vi "HFRR ADV v07.vi"() -> ()   [LabVIEW 2025] (continued)
                frame 81 {
                  n3117 = property on="Air Temperature  ( °C )" class="XYGraph (strict)"("Y Scale.Name Label.Text"=w4156) -> ()  [unwired: 2 in, 2 out]
                }
                frame 82 {
                  n3118 = local write "S 84"(w4157) -> ()
                }
                frame 83 {
                  n3119 = local write "S 85"(w4158) -> ()
                }
                frame 84 {
                  n3120 = local write "S 86"(w4159) -> ()
                }
                frame 85 {
                  n3121 = local write "S 87"(w4160) -> ()
                }
                frame 86 {
                  n3122 = local write "S 88"(w4161) -> ()
                }
                frame 87 {
                }
                frame 88 {
                  n3123 = local write "S 90"(w4163) -> ()
                }
                frame 89 {
                  n3124 = local write "S 91"(w4164) -> ()
                }
                frame 90 {
                  n3125 = local write "S 92"(w4165) -> ()
                }
                frame 91 {
                  n3126 = local write "S 93"(w4166) -> ()
                }
                frame 92 {
                  n3127 = local write "S 94"(w4167) -> ()
                }
                frame 93 {
                  n3128 = local write "S 95"(w4168) -> ()
                }
                frame 94 {
                  n3129 = local write "S 96"(w4169) -> ()
                }
                frame 95 {
                  n3130 = local write "S 97"(w4170) -> ()
                }
                frame 96 {
                  n3131 = local write "S 98"(w4171) -> ()
                }
                frame 97 {
                  n3132 = local write "S 99"(w4172) -> ()
                }
                frame 98 {
                  n3133 = local write "S 100"(w4173) -> ()
                }
                frame 99 {
                  n3134 = local write "S 101"(w4174) -> ()
                }
                frame 100 {
                  n3135 = local write "S 102"(w4175) -> ()
                }
                frame 101 {
                  n3136 = local write "S 103"(w4176) -> ()
                }
                frame 102 {
                  n3137 = local write "S 104"(w4177) -> ()
                }
                frame 103 {
                  n3138 = local write "S 105"(w4178) -> ()
                }
                frame 104 {
                  n3139 = local write "S 106"(w4179) -> ()
                }
                frame 105 {
                }
                frame 106 {
                  n3140 = property on="OK Button 17" class="Bool (strict)"("Boolean Text.Text"=w4180) -> ()  [unwired: 2 in, 2 out]
                }
                frame 107 {
                  n3141 = property on="OK Button 16" class="Bool (strict)"("Boolean Text.Text"=w4181) -> ()  [unwired: 2 in, 2 out]
                }
                frame 108 {
                  n3142 = property on="TITTLE" class="Str"("Caption.Text"=w4182) -> ()  [unwired: 2 in, 2 out]
                }
                frame 109 {
                  "String 30" <- w4183
                }
                frame 110 {
                  n3143 = property on="Test Date" class="Str"("Caption.Text"=w4184) -> ()  [unwired: 2 in, 2 out]
                  "String 31" <- w4184
                }
                frame 111 {
                  n3144 = property on="Sample ID" class="Str"("Caption.Text"=w4185) -> ()  [unwired: 2 in, 2 out]
                  "String 32" <- w4185
                }
                frame 112 {
                  n3145 = property on="Tested by" class="Str"("Caption.Text"=w4186) -> ()  [unwired: 2 in, 2 out]
                  "String 33" <- w4186
                }
                frame 113 {
                  n3146 = property on="System Configured Printers 2" class="Arr (strict)"("Caption.Text"=w4187) -> ()  [unwired: 2 in, 2 out]
                }
                frame 114 {
                  n3147 = property on="Selected Printer" class="Str"("Caption.Text"=w4188) -> ()  [unwired: 2 in, 2 out]
                }
                frame 115 {
                  n3148 = property on="Select Printer 3" class="DigNum (strict)"("Caption.Text"=w4189) -> ()  [unwired: 2 in, 2 out]
                }
                frame 116 {
                  n3149 = property on="Print" class="Bool (strict)"("Boolean Text.Text"=w4190) -> ()  [unwired: 2 in, 2 out]
                }
                frame 117 {
                  "String 41" <- w4191
                }
                frame 118 {
                  n3150 = property on="tested by" class="Str"("Caption.Text"=w4192) -> ()  [unwired: 2 in, 2 out]
                }
                frame 119 {
                }
                frame 120 {
                  n3151 = property on="Export" class="Bool (strict)"("Boolean Text.Text"=w4193) -> ()  [unwired: 2 in, 2 out]
                }
                frame 121 {
                  n3152 = property on="TEMP INTERCEPT:" class="DigNum (strict)"("Caption.Text"=w4194) -> ()  [unwired: 2 in, 2 out]
                }
                frame 122 {
                  n3153 = property on="AIR TEMP INTERCEPT:" class="DigNum (strict)"("Caption.Text"=w4195) -> ()  [unwired: 2 in, 2 out]
                }
                frame 123 {
                  n3154 = property on="Select File Type" class="Enum (strict)"("Caption.Text"=w4196) -> ()  [unwired: 2 in, 2 out]
                }
                frame 124 {
                  n3155 = property on="s.NO" class="Str"("Caption.Text"=w4197) -> ()  [unwired: 2 in, 2 out]
                  "String 45" <- w4197
                }
                frame 125 {
                  n3156 = property on="trip1 8" class="Bool (strict)"("Boolean Text.Text"=w4198) -> ()  [unwired: 2 in, 2 out]
                }
                frame 126, Default {
                }
              }
            }
          }
          frame #1 {
            w4206 = TRUE ("Visible")
            n3157 = local read "S 91"() -> (w4223:string)
            n3158 = local read "S 90"() -> (w4222:string)
            n3159 = local read "S 88"() -> (w4221:string)
            n3160 = property on="File Path" class="Path"("Caption.Text"=w4222) -> ()  [unwired: 2 in, 2 out]
            n3161 = property on="SrvM CP" class="Bool (strict)"("Boolean Text.Text"=w4221) -> ()  [unwired: 2 in, 2 out]
            n3162 = local read "S 71"() -> (w4216:string)
            n3163 = local read "S 86"() -> (w4218:string)
            n3164 = local read "S 85"() -> (w4219:string)
            n3165 = local read "S 87"() -> (w4217:string)
            n3166 = local read "S 84"() -> (w4220:string)
            n3167 = local read "S 103"() -> (w4205:string)
            n3168 = local read "S 104"() -> (w4204:string)
            n3169 = property on="ENTER THE NEW PASSWORD" class="Str"("Caption.Text"=w4217) -> ()  [unwired: 2 in, 2 out]
            n3170 = property on="Password" class="Str"("Caption.Text"=w4219) -> ()  [unwired: 2 in, 2 out]
            n3171 = property on="ENTER CURRENT PASSWORD" class="Str"("Caption.Text"=w4218) -> ()  [unwired: 2 in, 2 out]
            n3172 = property on="EDIT" class="Bool (strict)"("Boolean Text.Text"=w4216) -> ()  [unwired: 2 in, 2 out]
            n3173 = property on="SAVE" class="Bool (strict)"("Boolean Text.Text"=w4220) -> ()  [unwired: 2 in, 2 out]
            n3174 = Build Array(w4205, w4204) -> (w4203:string[])
            n3175 = property on="Heater Button" class="Bool (strict)"("Strings [4]"=w4203) -> ()  [unwired: 2 in, 2 out]
            n3176 = property on="CH-HUMIDITY WET" class="DigNum (strict)"("Caption.Size to Text?"=w4206) -> ()  [unwired: 2 in, 2 out]
            n3177 = property on="CH-HUMIDITY DRY" class="DigNum (strict)"("Caption.Size to Text?"=w4206) -> ()  [unwired: 2 in, 2 out]
            n3178 = property on="CH-POWER -" class="DigNum (strict)"("Caption.Size to Text?"=w4206) -> ()  [unwired: 2 in, 2 out]
            n3179 = property on="CH-HEATER" class="DigNum (strict)"("Caption.Size to Text?"=w4206) -> ()  [unwired: 2 in, 2 out]
            n3180 = property on="CH-POWER +" class="DigNum (strict)"("Caption.Size to Text?"=w4206) -> ()  [unwired: 2 in, 2 out]
            n3181 = local read "S 92"() -> (w4215:string)
            n3182 = local read "S 93"() -> (w4214:string)
            n3183 = local read "S 105"() -> (w4201:string)
            n3184 = local read "S 106"() -> (w4200:string)
            n3185 = Build Array(w4215, w4214) -> ()  [unwired: 1 out]
            n3186 = Build Array(w4201, w4200) -> (w4202:string[])
            n3187 = local read "S 95"() -> (w4212:string)
            n3188 = local read "S 94"() -> (w4213:string)
            n3189 = local read "bs"() -> (w4228:string)
            n3190 = local read "as"() -> (w4229:string)
            n3191 = property on="Humidity" class="Bool (strict)"("Strings [4]"=w4202) -> ()  [unwired: 2 in, 2 out]
            n3192 = Concatenate Strings(w4228, "\r", w4229) -> ()  [unwired: 1 out]
            n3193 = property on="STROKE GAIN :" class="DigNum (strict)"("Caption.Text"=w4212) -> ()  [unwired: 2 in, 2 out]
            n3194 = property on="DISPLACEMENT :" class="DigNum (strict)"("Caption.Text"=w4213) -> ()  [unwired: 2 in, 2 out]
            n3195 = property on="Rh After" class="DigNum (strict)"("Caption.Size to Text?"=TRUE ("Caption.Size to Text")) -> ()  [unwired: 2 in, 2 out]
            n3196 = local read "S 48"() -> (w4252:string)
            n3197 = local read "S 50"() -> (w4250:string)
            n3198 = local read "S 51"() -> (w4249:string)
            n3199 = local read "S 49"() -> (w4251:string)
            n3200 = local read "S 52"() -> (w4248:string)
            n3201 = local read "as"() -> (w4233:string)
            n3202 = local read "bs"() -> (w4234:string)
            n3203 = local read "S 56"() -> (w4247:string)
            n3204 = local read "S 57"() -> (w4246:string)
            n3205 = local read "S 58"() -> (w4245:string)
            n3206 = local read "S 59"() -> (w4244:string)
            n3207 = property on="OPEN" class="Bool (strict)"("Boolean Text.Text"=w4248) -> ()  [unwired: 2 in, 2 out]
            n3208 = property on="OPEN 1" class="Bool (strict)"("Boolean Text.Text"=w4252) -> ()  [unwired: 2 in, 2 out]
            n3209 = property on="OPEN 2" class="Bool (strict)"("Boolean Text.Text"=w4251) -> ()  [unwired: 2 in, 2 out]
            n3210 = property on="OPEN 3" class="Bool (strict)"("Boolean Text.Text"=w4250) -> ()  [unwired: 2 in, 2 out]
            n3211 = property on="OPEN 4" class="Bool (strict)"("Boolean Text.Text"=w4249) -> ()  [unwired: 2 in, 2 out]
            n3212 = Concatenate Strings(w4234, "\r", w4233) -> ()  [unwired: 1 out]
            n3213 = local read "S 102"() -> (w4207:string)
            n3214 = property on="КОФ1" class="DigNum (strict)"("Caption.Text"=w4247) -> ()  [unwired: 2 in, 2 out]
            n3215 = local read "S 98"() -> (w4211:string)
            n3216 = local read "S 99"() -> (w4210:string)
            n3217 = local read "S 100"() -> (w4209:string)
            n3218 = local read "S 101"() -> (w4208:string)
            n3219 = property on="КОФ2" class="DigNum (strict)"("Caption.Text"=w4246) -> ()  [unwired: 2 in, 2 out]
            n3220 = property on="КОФ3" class="DigNum (strict)"("Caption.Text"=w4245) -> ()  [unwired: 2 in, 2 out]
            n3221 = property on="КОФ4" class="DigNum (strict)"("Caption.Text"=w4244) -> ()  [unwired: 2 in, 2 out]
            n3222 = local read "bs"() -> (w4232:string)
            n3223 = local read "as"() -> (w4231:string)
            n3224 = property on="CH-POWER +" class="DigNum (strict)"("Caption.Text"=w4211) -> ()  [unwired: 2 in, 2 out]
            n3225 = property on="CH-POWER -" class="DigNum (strict)"("Caption.Text"=w4210) -> ()  [unwired: 2 in, 2 out]
            n3226 = property on="CH-HEATER" class="DigNum (strict)"("Caption.Text"=w4209) -> ()  [unwired: 2 in, 2 out]
            n3227 = property on="CH-HUMIDITY DRY" class="DigNum (strict)"("Caption.Text"=w4208) -> ()  [unwired: 2 in, 2 out]
            n3228 = property on="CH-HUMIDITY WET" class="DigNum (strict)"("Caption.Text"=w4207) -> ()  [unwired: 2 in, 2 out]
            n3229 = local read "S 60"() -> (w4243:string)
            n3230 = local read "S 54"() -> (w4253:string)
            n3231 = Concatenate Strings(w4232, "\r", w4231) -> ()  [unwired: 1 out]
            n3232 = Concatenate Strings(w4253, w4243) -> ()  [unwired: 1 out]
            n3233 = local read "S 77"() -> (→"String 43":string)
            n3234 = local read "S 76"() -> (w4226:string)
            n3235 = local read "S 78"() -> (w4225:string)
            n3236 = local read "S 71"() -> (w4237:string)
            n3237 = local read "S 66"() -> (w4242:string)
            n3238 = local read "S 67"() -> (w4241:string)
            n3239 = local read "S 68"() -> (w4240:string)
            n3240 = local read "S 69"() -> (w4239:string)
            n3241 = local read "S 70"() -> (w4238:string)
            n3242 = property on="AIR TEMP" class="DigNum (strict)"("Caption.Text"=w4225) -> ()  [unwired: 2 in, 2 out]
            n3243 = property on="Set Strk" class="DigNum (strict)"("Caption.Text"=w4226) -> ()  [unwired: 2 in, 2 out]
            n3244 = property on="FRIC. FORCE :" class="DigNum (strict)"("Caption.Text"=w4242) -> ()  [unwired: 2 in, 2 out]
            n3245 = property on="TEMPERATURE :" class="DigNum (strict)"("Caption.Text"=w4241) -> ()  [unwired: 2 in, 2 out]
            n3246 = property on="SPEED OUT:" class="DigNum (strict)"("Caption.Text"=w4240) -> ()  [unwired: 2 in, 2 out]
            n3247 = property on="AIR TEMPERATURE :" class="DigNum (strict)"("Caption.Text"=w4239) -> ()  [unwired: 2 in, 2 out]
            n3248 = property on="HUMIDITY:" class="DigNum (strict)"("Caption.Text"=w4238) -> ()  [unwired: 2 in, 2 out]
            n3249 = property on="EDIT" class="Bool (strict)"("Boolean Text.Text"=w4237) -> ()  [unwired: 2 in, 2 out]
            n3250 = local read "S 79"() -> (w4224:string)
          }
          frame #2 {
          }
        }
        n3251 = local write "Lan flag"(10.0 ("Lan flag")) -> ()
      }
      frame Enabled {
      }
    }
    n3252 = Wait (ms)(milliseconds to wait=u32 2000) -> ()  [unwired: 1 out]
    n3253 = local read "Quit"() -> (w4027:bool)
  }
  n3254 = disable-structure shown="Disabled" {
    frame Disabled {
      n3255 = while {
        tunnel: [w4255] -> _
        i -> [w4255]
        stop <- w4254 continue-if-true
        n3256 = Wait (ms)(milliseconds to wait=u32 50) -> ()  [unwired: 1 out]
        n3257 = stacked-sequence {
          frame #0 {
            # "Controls Text color"
            # "Controls BG color"
            n3258 = property on="FILE" class="Str"("Text.Text Colors:Text Color"="SC  Text") -> ()  [unwired: 2 in, 2 out]
            n3259 = property on="Fuel Discription :" class="Str"("Text.Text Colors:Text Color"="SC  Text") -> ()  [unwired: 2 in, 2 out]
            n3260 = property on="tested by" class="Str"("Text.Text Colors:Text Color"="SC  Text") -> ()  [unwired: 2 in, 2 out]
            n3261 = property on="Remarks :" class="Str"("Text.Text Colors:Text Color"="SC  Text") -> ()  [unwired: 2 in, 2 out]
            n3262 = property class="DigNum (strict)"("Numeric Text.Text Colors:BG Color"="NC BG") -> ()  [unwired: 2 in, 2 out]
            n3263 = property class="DigNum (strict)"("Numeric Text.Text Colors:BG Color"="NC BG") -> ()  [unwired: 2 in, 2 out]
            n3264 = property class="DigNum (strict)"("Numeric Text.Text Colors:BG Color"="NC BG") -> ()  [unwired: 2 in, 2 out]
            n3265 = property class="DigNum (strict)"("Numeric Text.Text Colors:BG Color"="NC BG") -> ()  [unwired: 2 in, 2 out]
            n3266 = property class="DigNum (strict)"("Numeric Text.Text Colors:BG Color"="NC BG") -> ()  [unwired: 2 in, 2 out]
            n3267 = property class="DigNum (strict)"("Numeric Text.Text Colors:BG Color"="NC BG") -> ()  [unwired: 2 in, 2 out]
            n3268 = property class="DigNum (strict)"("Numeric Text.Text Colors:BG Color"="NC BG") -> ()  [unwired: 2 in, 2 out]
            n3269 = property class="DigNum (strict)"("Numeric Text.Text Colors:BG Color"="NC BG") -> ()  [unwired: 2 in, 2 out]
            n3270 = property class="DigNum (strict)"("Numeric Text.Text Colors:BG Color"="NC BG") -> ()  [unwired: 2 in, 2 out]
            n3271 = property class="DigNum (strict)"("Numeric Text.Text Colors:BG Color"="NC BG") -> ()  [unwired: 2 in, 2 out]
            n3272 = property class="DigNum (strict)"("Numeric Text.Text Colors:BG Color"="NC BG") -> ()  [unwired: 2 in, 2 out]
            n3273 = property class="DigNum (strict)"("Numeric Text.Text Colors:BG Color"="NC BG") -> ()  [unwired: 2 in, 2 out]
            n3274 = property on="FILE" class="Str"("Text.Text Colors:BG Color"="SC BG 3") -> ()  [unwired: 2 in, 2 out]
            n3275 = property on="Fuel Discription :" class="Str"("Text.Text Colors:BG Color"="SC BG 3") -> ()  [unwired: 2 in, 2 out]
            n3276 = property on="tested by" class="Str"("Text.Text Colors:BG Color"="SC BG 3") -> ()  [unwired: 2 in, 2 out]
            n3277 = property on="Remarks :" class="Str"("Text.Text Colors:BG Color"="SC BG 3") -> ()  [unwired: 2 in, 2 out]
            n3278 = property class="DigNum (strict)"("Numeric Text.Text Colors:Text Color"="NC Text") -> ()  [unwired: 2 in, 2 out]
            n3279 = property class="DigNum (strict)"("Numeric Text.Text Colors:Text Color"="NC Text") -> ()  [unwired: 2 in, 2 out]
            n3280 = property class="DigNum (strict)"("Numeric Text.Text Colors:Text Color"="NC Text") -> ()  [unwired: 2 in, 2 out]
            n3281 = property class="DigNum (strict)"("Numeric Text.Text Colors:Text Color"="NC Text") -> ()  [unwired: 2 in, 2 out]
            n3282 = property class="DigNum (strict)"("Numeric Text.Text Colors:Text Color"="NC Text") -> ()  [unwired: 2 in, 2 out]
            n3283 = property class="DigNum (strict)"("Numeric Text.Text Colors:Text Color"="NC Text") -> ()  [unwired: 2 in, 2 out]
            n3284 = property class="DigNum (strict)"("Numeric Text.Text Colors:Text Color"="NC Text") -> ()  [unwired: 2 in, 2 out]
            n3285 = property class="DigNum (strict)"("Numeric Text.Text Colors:Text Color"="NC Text") -> ()  [unwired: 2 in, 2 out]
            n3286 = property class="DigNum (strict)"("Numeric Text.Text Colors:Text Color"="NC Text") -> ()  [unwired: 2 in, 2 out]
            n3287 = property class="DigNum (strict)"("Numeric Text.Text Colors:Text Color"="NC Text") -> ()  [unwired: 2 in, 2 out]
            n3288 = property class="DigNum (strict)"("Numeric Text.Text Colors:Text Color"="NC Text") -> ()  [unwired: 2 in, 2 out]
            n3289 = property class="DigNum (strict)"("Numeric Text.Text Colors:Text Color"="NC Text") -> ()  [unwired: 2 in, 2 out]
            n3290 = property class="DigNum (strict)"("Numeric Text.Text Colors:Text Color"="NI Text  2") -> ()  [unwired: 2 in, 2 out]
            n3291 = property class="DigNum (strict)"("Numeric Text.Text Colors:Text Color"="NI Text  2") -> ()  [unwired: 2 in, 2 out]
            n3292 = property class="DigNum (strict)"("Numeric Text.Text Colors:Text Color"="NI Text  2") -> ()  [unwired: 2 in, 2 out]
            n3293 = property class="DigNum (strict)"("Numeric Text.Text Colors:Text Color"="NI Text  2") -> ()  [unwired: 2 in, 2 out]
            n3294 = property class="DigNum (strict)"("Numeric Text.Text Colors:Text Color"="NI Text  2") -> ()  [unwired: 2 in, 2 out]
            n3295 = property class="DigNum (strict)"("Numeric Text.Text Colors:Text Color"="NI Text  2") -> ()  [unwired: 2 in, 2 out]
            n3296 = property class="DigNum (strict)"("Numeric Text.Text Colors:Text Color"="NI Text  2") -> ()  [unwired: 2 in, 2 out]
            n3297 = property class="DigNum (strict)"("Numeric Text.Text Colors:Text Color"="NI Text  2") -> ()  [unwired: 2 in, 2 out]
            n3298 = property class="DigNum (strict)"("Numeric Text.Text Colors:Text Color"="NI Text  2") -> ()  [unwired: 2 in, 2 out]
            n3299 = property class="DigNum (strict)"("Numeric Text.Text Colors:Text Color"="NI Text  2") -> ()  [unwired: 2 in, 2 out]
            n3300 = property class="DigNum (strict)"("Numeric Text.Text Colors:Text Color"="NI Text  2") -> ()  [unwired: 2 in, 2 out]
            n3301 = property class="DigNum (strict)"("Numeric Text.Text Colors:Text Color"="NI Text  2") -> ()  [unwired: 2 in, 2 out]
            n3302 = property class="DigNum (strict)"("Numeric Text.Text Colors:Text Color"="NI Text  2") -> ()  [unwired: 2 in, 2 out]
            n3303 = property class="DigNum (strict)"("Numeric Text.Text Colors:Text Color"="NI Text  2") -> ()  [unwired: 2 in, 2 out]
            n3304 = property class="DigNum (strict)"("Numeric Text.Text Colors:Text Color"="NI Text  2") -> ()  [unwired: 2 in, 2 out]
            n3305 = property on="Coefficient Of Friction" class="XYGraph (strict)"("Plot Area:Colors:FG Color"="GFG  2", "Plot Area:Colors:BG Color"="GBG   2") -> ()  [unwired: 2 in, 2 out]
            n3306 = property on="Humidity ( %RH )" class="XYGraph (strict)"("Plot Area:Colors:FG Color"="GFG  2", "Plot Area:Colors:BG Color"="GBG   2") -> ()  [unwired: 2 in, 2 out]
            n3307 = property on="Air Temperature  ( °C )" class="XYGraph (strict)"("Plot Area:Colors:FG Color"="GFG  2", "Plot Area:Colors:BG Color"="GBG   2") -> ()  [unwired: 2 in, 2 out]
            n3308 = property on="Sample Temperature ( °C )" class="XYGraph (strict)"("Plot Area:Colors:FG Color"="GFG  2", "Plot Area:Colors:BG Color"="GBG   2") -> ()  [unwired: 2 in, 2 out]
            n3309 = property class="DigNum (strict)"("Numeric Text.Text Colors:BG Color"="NI BG 2") -> ()  [unwired: 2 in, 2 out]
            n3310 = property class="DigNum (strict)"("Numeric Text.Text Colors:BG Color"="NI BG 2") -> ()  [unwired: 2 in, 2 out]
            n3311 = property class="DigNum (strict)"("Numeric Text.Text Colors:BG Color"="NI BG 2") -> ()  [unwired: 2 in, 2 out]
            n3312 = property class="DigNum (strict)"("Numeric Text.Text Colors:BG Color"="NI BG 2") -> ()  [unwired: 2 in, 2 out]
            n3313 = property class="DigNum (strict)"("Numeric Text.Text Colors:BG Color"="NI BG 2") -> ()  [unwired: 2 in, 2 out]
            n3314 = property class="DigNum (strict)"("Numeric Text.Text Colors:BG Color"="NI BG 2") -> ()  [unwired: 2 in, 2 out]
            n3315 = property class="DigNum (strict)"("Numeric Text.Text Colors:BG Color"="NI BG 2") -> ()  [unwired: 2 in, 2 out]
            n3316 = property class="DigNum (strict)"("Numeric Text.Text Colors:BG Color"="NI BG 2") -> ()  [unwired: 2 in, 2 out]
            n3317 = property class="DigNum (strict)"("Numeric Text.Text Colors:BG Color"="NI BG 2") -> ()  [unwired: 2 in, 2 out]
            n3318 = property class="DigNum (strict)"("Numeric Text.Text Colors:BG Color"="NI BG 2") -> ()  [unwired: 2 in, 2 out]
            n3319 = property class="DigNum (strict)"("Numeric Text.Text Colors:BG Color"="NI BG 2") -> ()  [unwired: 2 in, 2 out]
            n3320 = property class="DigNum (strict)"("Numeric Text.Text Colors:BG Color"="NI BG 2") -> ()  [unwired: 2 in, 2 out]
            n3321 = property class="DigNum (strict)"("Numeric Text.Text Colors:BG Color"="NI BG 2") -> ()  [unwired: 2 in, 2 out]
            n3322 = property class="DigNum (strict)"("Numeric Text.Text Colors:BG Color"="NI BG 2") -> ()  [unwired: 2 in, 2 out]
            n3323 = property class="DigNum (strict)"("Numeric Text.Text Colors:BG Color"="NI BG 2") -> ()  [unwired: 2 in, 2 out]
            n3324 = property class="Bool"("Colors [4]"="Boolean BC T & BG") -> ()  [unwired: 2 in, 2 out]
            n3325 = property on="Save & Continue" class="Bool (strict)"("Colors [4]"="Boolean BC T & BG") -> ()  [unwired: 2 in, 2 out]
            n3326 = property on="Heater Button" class="Bool (strict)"("Colors [4]"="Boolean BC T & BG") -> ()  [unwired: 2 in, 2 out]
            n3327 = property class="Bool"("Colors [4]"="Boolean BC T & BG") -> ()  [unwired: 2 in, 2 out]
            n3328 = property on="Humidity" class="Bool (strict)"("Colors [4]"="Boolean BC T & BG") -> ()  [unwired: 2 in, 2 out]
            n3329 = property class="Bool (strict)"("Colors [4]"="Boolean BC T & BG") -> ()  [unwired: 2 in, 2 out]
            n3330 = property on="RUN" class="Bool (strict)"("Colors [4]"="Boolean BC T & BG") -> ()  [unwired: 2 in, 2 out]
            n3331 = property on="trip1 8" class="Bool (strict)"("Colors [4]"="Boolean BC T & BG") -> ()  [unwired: 2 in, 2 out]
            n3332 = property class="Bool"("Colors [4]"="Boolean BC T & BG") -> ()  [unwired: 2 in, 2 out]
            n3333 = property class="Bool (strict)"("Colors [4]"="Boolean BC T & BG") -> ()  [unwired: 2 in, 2 out]
            n3334 = property on="OPEN 1" class="Bool (strict)"("Colors [4]"="Boolean BC T & BG 2") -> ()  [unwired: 2 in, 2 out]
            n3335 = property on="OPEN 2" class="Bool (strict)"("Colors [4]"="Boolean BC T & BG 2") -> ()  [unwired: 2 in, 2 out]
            n3336 = property on="OPEN 3" class="Bool (strict)"("Colors [4]"="Boolean BC T & BG 2") -> ()  [unwired: 2 in, 2 out]
            n3337 = property on="OPEN 4" class="Bool (strict)"("Colors [4]"="Boolean BC T & BG 2") -> ()  [unwired: 2 in, 2 out]
            n3338 = property on="OPEN" class="Bool (strict)"("Colors [4]"="Boolean BC T & BG 2") -> ()  [unwired: 2 in, 2 out]
            n3339 = property on="rstv2" class="Bool"("Colors [4]"="Boolean BC T & BG 2") -> ()  [unwired: 2 in, 2 out]
            n3340 = property on="RST CP" class="Bool"("Colors [4]"="Boolean BC T & BG 2") -> ()  [unwired: 2 in, 2 out]
            n3341 = property on="RSTV1 3" class="Bool"("Colors [4]"="Boolean BC T & BG 2") -> ()  [unwired: 2 in, 2 out]
            n3342 = property on="RSTV1 2" class="Bool"("Colors [4]"="Boolean BC T & BG 2") -> ()  [unwired: 2 in, 2 out]
          }
          frame #1 {
          }
        }
        n3343 = local read "Quit"() -> (w4254:bool)
      }
    }
    frame Enabled {
    }
  }
  n3344 = while {
    shift-right: [w4272] -> _
    shift-left: _ -> [w4273]
    shift-right: [w4270] -> _
    shift-left: T16 {"Read Heave and Surge"="", "Bytes at Heave Port"=0.0, "Heave and Surge COM Port:"="COM9", "Com Port 2"="COM7", "Residual Due"="", "Heave COM Status 2"=TRUE, "Heave COM Status"=TRUE, "Port 2"=TRUE, "Sway PPR"=6400.0, "Surge PPR"=6400.0, "Heave PPR"=6400.0, "Sway Pitch"=2.0, "Surge Pitch"=3.0, "Heave Pitch"=4.0, "Sway Pulses/mm"=320.0, "Surge Pulses/mm"=1600.0, "Heave Pulses/mm"=1600.0, "inner loop"=0.0, "Read Heave and Surge 2"="", "String 36"="", "Write S"=FALSE, "WriteCC1"=[""], "Heave COM Loop"=0, "LastCom"="", "EXIT"=FALSE, "Error Heave"={"status"=TRUE, "code"=-1073807343, "source"=""}} -> [w4269]
    shift-right: [w4267] -> _
    shift-left: enum16{"init", "MAIN", "Panel Close"}."init" -> [w4268]
    stop <- w4271 stop-if-true
    n3345 = case shown="\"init\"" w4268 {
      tunnel: w4273 -> [w4287 w4302 w4372 w4374]
      tunnel: [w4281 w4320 w4372 w4374] -> w4272
      tunnel: [_ _ TRUE _] -> w4271
      tunnel: [w4277 w4317 w4370 w4373] -> w4270
      tunnel: w4269 -> [w4284 w4301 w4370 w4373]
      tunnel: [enum16{"init", "MAIN", "Panel Close"}."MAIN" w4295 _ _] -> w4267
      frame "init" {
        n3346 = Bundle By Name(cluster=w4284, "Heave and Surge COM Port:"="C3 :") -> (w4283:T16)
        n3347 = call "Instrument fgv.vi"("Enum"=T28."INIT", "error in (no error) 2"=w4287, "INPUT"=w4283) -> ("error"=w4285:errorcluster, "output"=w4280:T16)  [unwired: 6 in, 1 out]
        n3348 = case shown="No Error" w4285 {
          selector: w4285 -> [w4289 _]
          tunnel: [w4289 w4293] -> w4281
          tunnel: w4280 -> [w4288 w4291]
          tunnel: [w4288 w4290] -> w4278
          frame No Error {
          }
          frame Error {
            n3349 = call "Instrument fgv.vi"("Enum"=T28."ERROR INIT", "INPUT"=w4291) -> ("error"=w4294:errorcluster, "output"=w4290:T16)  [unwired: 7 in, 1 out]
            n3350 = call <vilib>:"Clear Errors.vi"("error in (no error)"=w4294) -> ("error out"=w4293:errorcluster)  [unwired: 5 in, 1 out]
          }
        }
        n3351 = local read "LastCom"() -> (w4276:string)
        n3352 = Unbundle By Name(w4278) -> ("Heave COM Status 2"=→"COM Status" →"Instrument Status":bool, "Error Heave"=→"Error":errorcluster)  [unwired: 1 out]
        n3353 = Bundle By Name(cluster=w4278, "LastCom"=w4276) -> (w4277:T16)
      }
      frame "MAIN" {
        n3354 = Unbundle By Name(w4301) -> ("Com Port 2"=w4322:refnum<visa-resource-name>)
        n3355 = local write "Com Port 4"(w4322) -> ()
        n3356 = local read "C3 :"() -> (w4299:refnum<visa-resource-name>)
        n3357 = Divide(x="Heave PPR", y="Heave Pitch") -> (x/y=→"Heave Pulses/mm":dbl)
        n3358 = Bundle By Name(cluster=w4301, "Heave and Surge COM Port:"=w4299) -> (w4300:T16)
        n3359 = Equal?(x=w4322, y=w4299) -> (x = y?=w4321:bool)
        n3360 = Divide(x="Sway PPR", y="Sway Pitch") -> (x/y=→"Sway Pulses/mm":dbl)
        n3361 = case shown="False" w4321 {
          tunnel: [w4326 w4343] -> w4320
          tunnel: w4302 -> [w4327 w4349]
          tunnel: w4300 -> [w4325 w4347]
          tunnel: [w4324 w4342] -> w4317
          frame False {
            n3362 = call <vilib>:"Clear Errors.vi"("error in (no error)"=w4327) -> ("error out"=w4323:errorcluster)  [unwired: 5 in, 1 out]
            n3363 = call "Instrument fgv.vi"("Enum"=T28."ERROR INIT", "error in (no error) 2"=w4323, "INPUT"=w4325) -> ("error"=w4329:errorcluster, "output"=w4324:T16)  [unwired: 6 in, 1 out]
            n3364 = call <vilib>:"Clear Errors.vi"("error in (no error)"=w4329) -> ("error out"=w4326:errorcluster)  [unwired: 5 in, 1 out]
          }
          frame True {
            n3365 = call "Instrument fgv.vi"("Enum"=T28."READ", "error in (no error) 2"=w4349, "INPUT"=w4347) -> ("error"=w4348:errorcluster, "output"=w4339:T16)  [unwired: 6 in, 1 out]
            n3366 = Bundle By Name(cluster=w4339, "String 36"="String 11") -> (w4338:T16)
            n3367 = case shown="True" "Write S" {
              selector: "Write S" -> [_ w4369]
              tunnel: w4348 -> [w4362 w4368]
              tunnel: [w4362 w4367] -> w4335
              tunnel: w4338 -> [w4361 w4364]
              tunnel: [w4361 w4363] -> w4334
              frame False {
              }
              frame True {
                n3368 = Not(x=w4369) -> (.not. x?=w4365:bool)
                n3369 = local write "Write S"(w4365) -> ()
                n3370 = call "Instrument fgv.vi"("Enum"=T28."MANUAL WRITE", "error in (no error) 2"=w4368, "INPUT"=w4364) -> ("error"=w4367:errorcluster, "output"=w4363:T16)  [unwired: 6 in, 1 out]
              }
            }
            n3371 = Array Size(array="WriteHumidity") -> (size(s)=w4332:i32)
            n3372 = Greater Than 0?(x=w4332) -> (x > 0?=w4330:bool)
            n3373 = call "Instrument fgv.vi"("Enum"=T28."WRITE", "error in (no error) 2"=w4335, "WriteCC1"="WriteHumidity", "INPUT"=w4334) -> ("error"=w4345:errorcluster, "WriteCC1 2"=w4333:string[], "output"=w4344:T16)  [unwired: 5 in]
            n3374 = case shown="True" w4330 {
              tunnel: w4333 -> [_ w4351]
              frame False {
              }
              frame True {
                n3375 = local write "WriteHumidity"(w4351) -> ()
              }
            }
            n3376 = case shown="Error" w4345 {
              selector: w4345 -> [w4352 w4355]
              tunnel: w4344 -> [w4353 w4360]
              tunnel: [w4353 w4359] -> w4342
              tunnel: [w4352 w4357] -> w4343
              frame No Error {
              }
              frame Error {
                n3377 = call <vilib>:"Clear Errors.vi"("error in (no error)"=w4355) -> ("error out"=w4354:errorcluster)  [unwired: 5 in, 1 out]
                n3378 = call "Instrument fgv.vi"("Enum"=T28."ERROR INIT", "error in (no error) 2"=w4354, "INPUT"=w4360) -> ("error"=w4358:errorcluster, "output"=w4359:T16)  [unwired: 6 in, 1 out]
                n3379 = call <vilib>:"Clear Errors.vi"("error in (no error)"=w4358) -> ("error out"=w4357:errorcluster)  [unwired: 5 in, 1 out]
              }
            }
            n3380 = Unbundle By Name(w4342) -> ("LastCom"=→"LastCom":string, "Read Heave and Surge"=→"Read Humidity":string)
          }
        }
        n3381 = Divide(x="Surge PPR", y="Surge Pitch") -> (x/y=→"Surge Pulses/mm":dbl)
        n3382 = Unbundle By Name(w4317) -> ("Heave COM Status 2"=w4319:bool, "Heave COM Status"=w4318:bool, "Error Heave"=w4315:errorcluster, "Bytes at Heave Port"=→"Bytes at Humidity Port":dbl)
        n3383 = Unbundle By Name(w4315) -> ("status"=→"Humidity Port":bool)
        n3384 = Not(x=w4318) -> (.not. x?=w4303:bool)
        n3385 = local write "Error"(w4315) -> ()
        n3386 = Not(x=w4319) -> (.not. x?=w4304:bool)
        n3387 = local write "Instrument Status"(w4303) -> ()
        n3388 = local write "COM Status"(w4304) -> ()
        n3389 = local read "Quit"() -> (w4296:bool)
        n3390 = Select(t=enum16{"init", "MAIN", "Panel Close"}."Panel Close", s=w4296, f=enum16{"init", "MAIN", "Panel Close"}."MAIN") -> (s? t:f=w4295:enum16{"init", "MAIN", "Panel Close"})
      }
      frame "Panel Close" {
      }
      frame Default {
      }
    }
  }
  n3391 = while {
    stop <- w4400 stop-if-true
    n3392 = local read "Read Humidity"() -> (w4381:string)
    n3393 = call <vilib>:"High Resolution Polling Wait.vi"("seconds to wait"=0.1) -> ()  [unwired: 10 in, 1 out]
    n3394 = Spreadsheet String To Array(delimiter (Tab)=",", format string="", spreadsheet string=w4381, array type (2D Dbl)=string[] []) -> (array=w4395:string[])
    n3395 = for {
      tunnel: w4395 -> [w4405] mode=indexing
      tunnel: string[] ["STATE;", "SET;", "RH;", "T;", "AMB_RH;", "AMB_T;", "PUMP;", "FAN_IN;", "FAN_OUT;", "DEHUM;", "CURRENT;", "STALL;"] -> [w4404] mode=indexing
      tunnel: [w4403] -> w4394 mode=indexing
      n3396 = Match Pattern(string=w4405, regular expression=w4404) -> (after substring=w4403:string)  [unwired: 1 in, 3 out]
    }
    n3397 = Index Array(array=w4394) -> (element #1=→"STATE :":string, element #2=→"SET :":string, element #3=w4383:string, element #4=→"T :":string, element #5=w4380:string, element #6=→"AMB_T :":string, element #7=→"PUMP :":string, element #8=→"FAN_IN :":string, element #9=→"FAN_OUT :":string, element #10=→"DEHUM :":string, element #11=→"CURRENT :":string, element #12=→"STALL :":string)  [unwired: 12 in]
    "RH :" <- w4383
    "AMB_RH :" <- w4380
    n3398 = Fract/Exp String To Number(string=w4383) -> (number=w4375:dbl)  [unwired: 3 in, 1 out]
    n3399 = Fract/Exp String To Number(string=w4380) -> (number=w4379:dbl)  [unwired: 3 in, 1 out]
    n3400 = local write "Ambient Humidity :"(w4379) -> ()
    n3401 = Equal?(x=w4375, y=0.0) -> (x = y?=w4377:bool)
    n3402 = case shown="True" w4377 {
      tunnel: [w4401 w4402] -> w4376
      tunnel: w4375 -> [w4401 _]
      frame False {
        (unwired) 0.0
        "Humidity temp" <- w4401
      }
      frame True {
        n3403 = local read "Humidity temp"() -> (w4402:dbl)
      }
    }
    "RH Numeric:" <- w4376
    n3404 = local read "Quit"() -> (w4400:bool)
  }
  n3405 = disable-structure shown="Disabled" {
    frame Disabled {
      n3406 = while {
        tunnel: [w4639] -> _
        i -> [w4639]
        stop <- w4636 stop-if-true
        n3407 = local read "powstat"() -> (w4637:bool)
        n3408 = case shown="True" w4637 {
          frame False {
          }
          frame True {
            n3409 = local read "RUN"() -> (w4640:bool)
            n3410 = case shown="True" w4640 {
              frame False {
                w4670 = 65.0 ("y")
                n3411 = local read "Set Hz"() -> (w4698:dbl)
                n3412 = local read "NORMAL LOAD"() -> (w4699:dbl)
                n3413 = Multiply(x=w4698, y=60.0) -> (x*y=w4705:dbl)
                n3414 = Multiply(x=1.2 ("y"), y=0.949) -> (x*y=w4674:dbl)
                n3415 = Multiply(x=1.2 ("y"), y=0.851) -> (x*y=w4673:dbl)
                n3416 = Multiply(x=1.2 ("y"), y=0.8166) -> (x*y=w4678:dbl)
                n3417 = local read "FF 2"() -> (w4697:dbl)
                n3418 = Absolute Value(x=w4705) -> (abs(x)=w4703:dbl)
                n3419 = case shown="13.." w4697 {
                  tunnel: [1 2 3] -> w4695
                  frame 0..10, Default {
                    # "Normal"
                  }
                  frame 11, 12 {
                  }
                  frame 13.. {
                  }
                }
                "FF STATE" <- w4695
                n3420 = local read "TEMP"() -> (w4658:dbl)
                n3421 = local read item#-1() -> (w4672)
                n3422 = Less?(x=w4672, y=w4678) -> (x < y?=w4675:bool)
                n3423 = In Range and Coerce(upper limit=w4674, x=w4672, lower limit=w4673) -> (In Range?=w4676:bool)  [unwired: 1 out]
                n3424 = case shown="3601.." w4703 {
                  tunnel: [1 2 3] -> w4701
                  frame 0..3000, Default {
                    # "Normal"
                  }
                  frame 3001..3600 {
                  }
                  frame 3601.. {
                  }
                }
                n3425 = case shown="11.." w4699 {
                  tunnel: [1 3] -> w4700
                  frame 1..10, Default {
                  }
                  frame 11.. {
                  }
                }
                "NL STATE" <- w4700
                n3426 = Multiply(x=1.2 ("y"), y=0.95) -> (x*y=w4688:dbl)
                n3427 = Multiply(x=w4670, y=0.954) -> (x*y=w4662:dbl)
                n3428 = Or(x=w4675, y=w4676) -> (x .or. y?=w4677:bool)
                n3429 = Greater Or Equal?(x=w4672, y=w4688) -> (x >= y?=w4685:bool)
                n3430 = Multiply(x=w4670, y=0.99) -> (x*y=w4659:dbl)
                n3431 = Greater Or Equal?(x=w4658, y=w4659) -> (x >= y?=w4664:bool)
                n3432 = Greater Or Equal?(x=w4658, y=w4662) -> (x >= y?=w4661:bool)
                n3433 = case shown="0, 1, Default" w4672 {
                  tunnel: [1 3] -> w4689
                  frame 0, 1, Default {
                  }
                  frame 2.. {
                  }
                }
                n3434 = case shown="True" w4685 {
                  tunnel: [1 3] -> w4690
                  frame False {
                  }
                  frame True {
                  }
                }
                n3435 = case shown="True" w4677 {
                  tunnel: [1 2] -> w4691
                  frame False {
                  }
                  frame True {
                  }
                }
                n3436 = case shown="..0" w4658 {
                  tunnel: [2 3 3 1] -> w4665
                  frame 61, 62 {
                  }
                  frame 63.. {
                  }
                  frame ..0 {
                  }
                  frame 10..60, Default {
                  }
                }
                n3437 = case shown="True" w4664 {
                  tunnel: [1 3] -> w4666
                  frame False {
                  }
                  frame True {
                  }
                }
                n3438 = case shown="True" w4661 {
                  tunnel: [1 2] -> w4667
                  frame False {
                  }
                  frame True {
                  }
                }
                n3439 = Number To Decimal String(number=w4701) -> (decimal integer string=w4702:string)  [unwired: 1 in]
                n3440 = Number To Decimal String(number=1) -> (decimal integer string=→"Air temp":string)  [unwired: 1 in]
                n3441 = Number To Decimal String(number=w4695) -> (decimal integer string=→"ff_st":string)  [unwired: 1 in]
                n3442 = local write "sp_st"(w4702) -> ()
                n3443 = Number To Decimal String(number=w4700) -> (decimal integer string=→"nl_st":string)  [unwired: 1 in]
                n3444 = Build Array(w4665, w4666, w4667) -> (w4668:i32[])
                n3445 = Build Array(w4689, w4690, w4691) -> (w4692:i32[])
                n3446 = Array Max & Min(array=w4668) -> (max value=w4669:i32)  [unwired: 3 out]
                n3447 = Array Max & Min(array=w4692) -> (max value=w4693:i32)  [unwired: 3 out]
                n3448 = Number To Decimal String(number=w4669) -> (decimal integer string=w4657:string)  [unwired: 1 in]
                n3449 = Number To Decimal String(number=w4693) -> (decimal integer string=→"Stroke Ln 2":string)  [unwired: 1 in]
                n3450 = local write "temp_st"(w4657) -> ()
              }
              frame True {
                w4755 = 65.0 ("y")
                # "Healthy -1\nWarning -2\nError -3"
                n3451 = local read "TEMP"() -> (w4766:dbl)
                n3452 = local read "NORMAL LOAD"() -> (w4770:dbl)
                n3453 = local read "Set Hz"() -> (w4768:dbl)
                n3454 = Multiply(x=1.2 ("y"), y=0.949) -> (x*y=w4750:dbl)
                n3455 = Multiply(x=1.2 ("y"), y=0.851) -> (x*y=w4751:dbl)
                n3456 = Multiply(x=1.2 ("y"), y=0.8166) -> (x*y=w4746:dbl)
                n3457 = Multiply(x=w4755, y=0.954) -> (x*y=w4762:dbl)
                n3458 = Multiply(x=w4755, y=0.99) -> (x*y=w4765:dbl)
                n3459 = Greater Or Equal?(x=w4766, y=w4765) -> (x >= y?=w4760:bool)
                n3460 = Multiply(x=w4768, y=60.0) -> (x*y=w4774:dbl)
                n3461 = Greater Or Equal?(x=w4766, y=w4762) -> (x >= y?=w4763:bool)
                n3462 = local read "FF 2"() -> (w4769:dbl)
                n3463 = local read item#-1() -> (w4752)
                n3464 = Less?(x=w4752, y=w4746) -> (x < y?=w4749:bool)
                n3465 = In Range and Coerce(upper limit=w4750, x=w4752, lower limit=w4751) -> (In Range?=w4748:bool)  [unwired: 1 out]
                n3466 = Absolute Value(x=w4774) -> (abs(x)=w4772:dbl)
                n3467 = case shown="63.." w4766 {
                  tunnel: [2 3 3 1] -> w4759
                  frame 61, 62 {
                  }
                  frame 63.. {
                  }
                  frame ..0 {
                  }
                  frame 10..60, Default {
                  }
                }
                n3468 = case shown="True" w4760 {
                  tunnel: [1 3] -> w4758
                  frame False {
                  }
                  frame True {
                  }
                }
                n3469 = case shown="True" w4763 {
                  tunnel: [1 2] -> w4757
                  frame False {
                  }
                  frame True {
                  }
                }
                n3470 = Multiply(x=1.2 ("y"), y=0.95) -> (x*y=w4736:dbl)
                n3471 = case shown="1..10, Default" w4770 {
                  tunnel: [1 3] -> w4777
                  frame 1..10, Default {
                  }
                  frame 11.. {
                  }
                }
                n3472 = case shown="0..10, Default" w4769 {
                  tunnel: [1 2 3] -> w4776
                  frame 0..10, Default {
                  }
                  frame 11, 12 {
                  }
                  frame 13.. {
                  }
                }
                n3473 = case shown="3601.." w4772 {
                  tunnel: [1 2 3] -> w4771
                  frame 0..3000, Default {
                    # "Normal"
                  }
                  frame 3001..3600 {
                  }
                  frame 3601.. {
                  }
                }
                n3474 = Or(x=w4749, y=w4748) -> (x .or. y?=w4747:bool)
                n3475 = Greater Or Equal?(x=w4752, y=w4736) -> (x >= y?=w4739:bool)
                n3476 = case shown="0, 1, Default" w4752 {
                  tunnel: [1 3] -> w4735
                  frame 0, 1, Default {
                  }
                  frame 2.. {
                  }
                }
                n3477 = case shown="True" w4739 {
                  tunnel: [1 3] -> w4734
                  frame False {
                  }
                  frame True {
                  }
                }
                n3478 = case shown="True" w4747 {
                  tunnel: [1 2] -> w4733
                  frame False {
                  }
                  frame True {
                  }
                }
                n3479 = Build Array(w4759, w4758, w4757) -> (w4756:i32[])
                n3480 = Number To Decimal String(number=w4771) -> (decimal integer string=→"sp_st":string)  [unwired: 1 in]
                n3481 = Array Max & Min(array=w4756) -> (max value=w4753:i32)  [unwired: 3 out]
                "TEMP STATE" <- w4753
                n3482 = Number To Decimal String(number=w4777) -> (decimal integer string=w4780:string)  [unwired: 1 in]
                n3483 = Number To Decimal String(number=w4776) -> (decimal integer string=w4778:string)  [unwired: 1 in]
                n3484 = Number To Decimal String(number=w4753) -> (decimal integer string=→"temp_st":string)  [unwired: 1 in]
                n3485 = Build Array(w4735, w4734, w4733) -> (w4732:i32[])
                n3486 = local write "nl_st"(w4780) -> ()
                n3487 = local write "ff_st"(w4778) -> ()
                n3488 = Number To Decimal String(number=1) -> (decimal integer string=w4775:string)  [unwired: 1 in]
                n3489 = Array Max & Min(array=w4732) -> (max value=w4731:i32)  [unwired: 3 out]
                n3490 = local write "Air temp"(w4775) -> ()
                n3491 = Number To Decimal String(number=w4731) -> (decimal integer string=w4730:string)  [unwired: 1 in]
                n3492 = local write "Stroke Ln 2"(w4730) -> ()
              }
            }
            n3493 = local read "Stroke Ln 2"() -> (w4642:string)
            n3494 = local read "ff_st"() -> (w4645:string)
            n3495 = local read "sp_st"() -> (w4646:string)
            n3496 = local read "nl_st"() -> (w4648:string)
            n3497 = local read "temp_st"() -> (w4647:string)
            n3498 = local read "Air temp"() -> (w4641:string)
            n3499 = Replace Array Subset(array="in", new element #1=w4648, index #1=1 ("index"), new element #2=w4645, index #2=2 ("index"), new element #3=w4647, index #3=3 ("index"), new element #4=w4646, index #4=4 ("index"), new element #5=w4642, index #5=5 ("index"), new element #6=w4641, index #6=6 ("index"), new element #7="Sensor State" ("new element/subarray"), index #7=0 ("index")) -> (→"out":string[])
          }
        }
        n3500 = Wait (ms)(milliseconds to wait=u32 10) -> ()  [unwired: 1 out]
        n3501 = local read "Quit"() -> (w4636:bool)
      }
      n3502 = while {
        stop <- w4611 stop-if-true
        n3503 = local read "run replace"() -> (w4613:bool)
        n3504 = Wait (ms)(milliseconds to wait=u32 100) -> ()  [unwired: 1 out]
        n3505 = Equal?(x="FLAG 2", y=0.0) -> (x = y?=w4614:bool)
        n3506 = case shown="True" w4614 {
          frame False {
          }
          frame True {
            n3507 = local write "FLAG 2"(100.0 ("FLAG 2")) -> ()
            n3508 = call <vilib>:"Read Characters From File.vi"("file path (dialog if empty)"=path "C:/LAB-IQ-NXT/WO 2449 TT.sig", "convert eol? (no:F)"=FALSE ("append to file? (new file:F)")) -> ("character string"=w4617:string)  [unwired: 4 in, 3 out]
            n3509 = call <vilib>:"Read Characters From File.vi"("file path (dialog if empty)"=path "C:/LAB-IQ-NXT/WO 2449 TRH.sig", "convert eol? (no:F)"=FALSE ("append to file? (new file:F)")) -> ("character string"=w4618:string)  [unwired: 4 in, 3 out]
            n3510 = Decimal String To Number(string=w4617) -> (number=w4619:i32)  [unwired: 2 in, 1 out]
            n3511 = local write "Total No. of Tests"(w4619) -> ()
            n3512 = Decimal String To Number(string=w4618) -> (number=w4622:i32)  [unwired: 2 in, 1 out]
            n3513 = local write "SEN.RUN HRS"(w4622) -> ()
          }
        }
        n3514 = case shown="True" w4613 {
          frame False {
          }
          frame True {
            n3515 = Equal?(x="FLAG 4", y=0.0) -> (x = y?=w4626:bool)
            n3516 = case shown="False" w4626 {
              frame False {
                n3517 = Get Date/Time In Seconds() -> (seconds since 1Jan1904=w4632:timestamp)
                n3518 = local read "START 3"() -> (w4630:dbl)
                n3519 = To Double Precision Float(number=w4632) -> (double precision float=w4631:dbl)
                n3520 = Subtract(x=w4631, y=w4630) -> (x-y=→"SENSOR TIME":dbl)
              }
              frame True {
                n3521 = Get Date/Time In Seconds() -> (seconds since 1Jan1904=w4634:timestamp)
                n3522 = local write "FLAG 4"(100.0 ("FLAG")) -> ()
                n3523 = To Double Precision Float(number=w4634) -> (double precision float=→"START 3":dbl)
              }
            }
          }
        }
        n3524 = local read "Quit"() -> (w4611:bool)
      }
      n3525 = while {
        shift-right: [w4411] -> _
        shift-left: _ -> [w4412]
        tunnel: [w4407] -> _
        i -> [w4407]
        stop <- w4406 stop-if-true
        n3526 = Wait (ms)(milliseconds to wait=u32 50 ("Refresh Rate (ms)")) -> ()  [unwired: 1 out]
        n3527 = local read "Json End Flg"() -> (w4408:bool)
        n3528 = Not(x="Upld AR 2") -> ()  [unwired: 1 out]
        n3529 = local read "Upld AR 2"() -> (w4409:bool)
        n3530 = call "Elapsed Time9"("Time Target (s)"="Sen.Upload Rate (s)", "Reset"=FALSE, "Auto Reset"=TRUE) -> ("Time has Elapsed"=w4418:bool)  [unwired: 9 in, 7 out]
        n3531 = Or(x=w4418, y=w4408) -> (x .or. y?=w4414:bool)
        n3532 = case shown="True" w4414 {
          frame False {
          }
          frame True {
            w4510 = "\"SensorName\":\"" ("string")
            w4480 = " \"},{"
            w4505 = "\",\"SensorState\":\""
            w4507 = "\",\"SensorModelNumber\":\"" ("string")
            w4506 = "\",\"SensorRuntimeHours\":\"" ("string")
            n3533 = local read "model num"() -> (w4504:string[])
            n3534 = local read "Sensor name"() -> (w4523:string[])
            n3535 = local read "run"() -> (w4494:string[])
            n3536 = local read "SENSOR TIME"() -> (w4450:dbl)
            n3537 = local read "out"() -> (w4443:string[])
            n3538 = local read "Total No. of Tests"() -> (w4448:dbl)
            n3539 = Select(t=60.0, s="Run test 3", f=3600.0) -> (s? t:f=w4458:dbl)
            n3540 = Index Array(array=w4504, index #1=1 ("index")) -> (element #1=w4503:string, element #2=w4502:string, element #3=w4501:string, element #4=w4500:string, element #5=w4499:string, element #6=w4498:string)  [unwired: 5 in]
            n3541 = Index Array(array=w4494, index #1=1 ("index")) -> (element #1=w4493:string, element #2=w4492:string, element #3=w4491:string, element #4=w4490:string, element #5=w4489:string, element #6=w4488:string)  [unwired: 5 in]
            n3542 = Index Array(array=w4523, index #1=1 ("index")) -> (element #1=w4522:string, element #2=w4521:string, element #3=w4520:string, element #4=w4519:string, element #5=w4509:string, element #6=w4508:string)  [unwired: 5 in]
            n3543 = Index Array(array=w4443, index #1=1 ("index")) -> (element #1=w4475:string, element #2=w4474:string, element #3=w4473:string, element #4=w4472:string, element #5=w4471:string, element #6=w4470:string)  [unwired: 5 in]
            n3544 = local read "SEN.RUN HRS"() -> (w4446:dbl)
            n3545 = Divide(x=w4450, y=w4458) -> (x/y=w4457:dbl)
            n3546 = Increment(x=w4457) -> (x+1=w4453:dbl)
            n3547 = Number To Decimal String(number=w4453) -> (decimal integer string=→"run hrs":string)  [unwired: 1 in]
            n3548 = Divide(x=w4446, y=3600.0 ("f")) -> (x/y=w4441:dbl)
            n3549 = Round To Nearest(number=w4441) -> (nearest integer value=w4439:dbl)
            n3550 = Number To Decimal String(number=w4439) -> (decimal integer string=w4440:string)  [unwired: 1 in]
            n3551 = Number To Decimal String(number=w4448) -> (decimal integer string=w4449:string)  [unwired: 1 in]
            n3552 = local read "Model No"() -> (w4454:string)
            n3553 = local read "UUID"() -> (w4549:string)
            n3554 = local read "Serial No"() -> (w4553:string)
            n3555 = local read "Secret Key"() -> (w4554:string)
            n3556 = Concatenate Strings("\",\"ModelNumber\":\"" ("string"), w4454) -> (w4455:string)
            n3557 = Concatenate Strings("\",\"MachineRuntimeCycles\":\"", w4449) -> (w4551:string)
            n3558 = Concatenate Strings("\",\"MachineRuntimeHours\":\"" ("string"), w4440) -> (w4558:string)
            n3559 = Concatenate Strings("\",\"MachineSerialNumber\":\"" ("string"), w4553) -> (w4557:string)
            n3560 = Concatenate Strings(w4506, w4493) -> (w4538:string)
            n3561 = Concatenate Strings(w4507, w4503) -> (w4537:string)
            n3562 = Concatenate Strings(w4505, w4475) -> (w4536:string)
            n3563 = Concatenate Strings(w4557, w4455, w4558, w4551) -> (w4560:string)
            n3564 = Concatenate Strings(w4506, w4492) -> (w4533:string)
            n3565 = Concatenate Strings(w4507, w4502) -> (w4534:string)
            n3566 = Concatenate Strings(w4506, w4491) -> (w4530:string)
            n3567 = Concatenate Strings(w4507, w4501) -> (w4529:string)
            n3568 = Concatenate Strings(w4505, w4474) -> (w4535:string)
            n3569 = Concatenate Strings(w4505, w4473) -> (w4528:string)
            n3570 = Concatenate Strings(w4506, w4490) -> (w4525:string)
            n3571 = Concatenate Strings(w4507, w4500) -> (w4526:string)
            n3572 = Concatenate Strings(w4505, w4472) -> (w4527:string)
            n3573 = Concatenate Strings(w4537, w4538, w4536) -> (w4539:string)
            n3574 = Concatenate Strings(w4506, w4489) -> (w4517:string)
            n3575 = Concatenate Strings(w4507, w4499) -> (w4516:string)
            n3576 = Concatenate Strings(w4506, w4488) -> (w4512:string)
            n3577 = Concatenate Strings(w4507, w4498) -> (w4513:string)
            n3578 = Concatenate Strings(w4505, w4471) -> (w4515:string)
            n3579 = Concatenate Strings(w4505, w4470) -> (w4514:string)
            n3580 = Concatenate Strings("{\"SecretKey\":\"", w4554, w4560, "\",\"UUID\" : \"", w4549, "\",\"SensorInformation\":", "[{" ("string")) -> (w4487:string)
            n3581 = Concatenate Strings(w4534, w4533, w4535) -> (w4532:string)
            n3582 = Concatenate Strings(w4529, w4530, w4528) -> (w4531:string)
            n3583 = Concatenate Strings(w4526, w4525, w4527) -> (w4524:string)
            n3584 = Concatenate Strings(w4516, w4517, w4515) -> (w4518:string)
            n3585 = Concatenate Strings(w4513, w4512, w4514) -> (w4511:string)
            n3586 = Concatenate Strings(w4510, w4522, w4539, w4480) -> (w4486:string)
            n3587 = Concatenate Strings(w4510, w4521, w4532, w4480) -> (w4485:string)
            n3588 = Concatenate Strings(w4510, w4520, w4531, w4480) -> (w4484:string)
            n3589 = Concatenate Strings(w4510, w4519, w4524, w4480) -> (w4483:string)
            n3590 = Concatenate Strings(w4510, w4509, w4518, w4480) -> (w4482:string)
            n3591 = Concatenate Strings(w4510, w4508, w4511, "\"}" ("string")) -> (w4481:string)
            n3592 = Concatenate Strings(w4487, w4486, w4485, w4484, w4483, w4482, w4481, "]}" ("string")) -> (w4478:string)
            n3593 = local read "SEN.RUN HRS"() -> (w4445:dbl)
            n3594 = disable-structure shown="Disabled" {
              frame Disabled {
                n3595 = local read "state"() -> (w4564:string[])
                n3596 = Delete From Array(array=w4564, index=0) -> (array with subset deleted=w4562:string[])  [unwired: 1 in, 1 out]
                n3597 = for {
                  N: 6 -> [_]
                  tunnel: w4562 -> [w4575] mode=indexing
                  tunnel: [w4574] -> w4561 mode=indexing
                  n3598 = Equal?(x=w4575, y="Warning") -> (x = y?=w4571:bool)
                  n3599 = Equal?(x=w4575, y="Healthy") -> (x = y?=w4568:bool)
                  n3600 = Select(t="2" ("y"), s=w4571, f="3" ("y")) -> (s? t:f=w4566:string)
                  n3601 = Select(t="1" ("y"), s=w4568, f=w4566) -> (s? t:f=w4574:string)
                }
